vi "Read menu reference.vi"(8 "error in (no error)":errorcluster, 11 "Waveform_Task in":refnum<class "Waveform_Task.lvclass">) -> (0 "error out":errorcluster, 2 "menu reference":refnum<k9>, 3 "Waveform_Task out":refnum<class "Waveform_Task.lvclass">)   [LabVIEW 2025, in "Waveform_Task.lvlib" / "Waveform_Task.lvclass"]
uses:
  Waveform_Task.lvclass
  Waveform_Task.lvclass/Waveform_Task.ctl
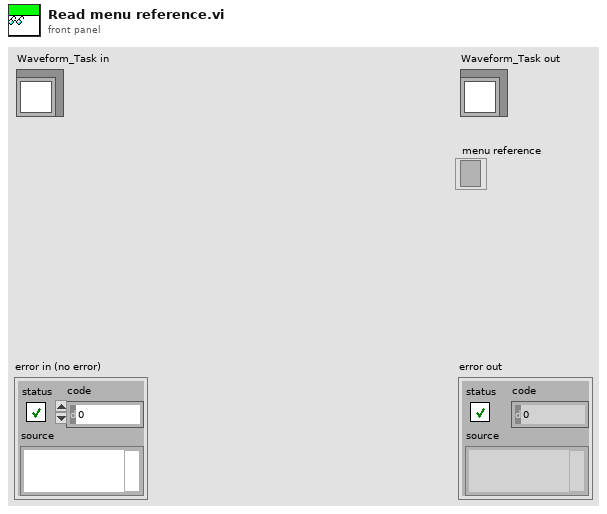
[diagram p1: front panel]
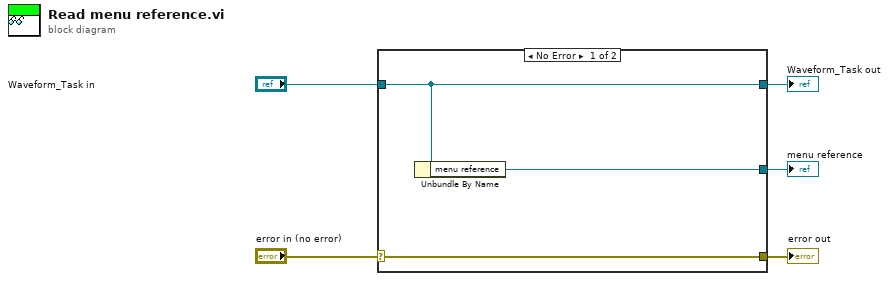
[diagram p0: block diagram]
diagram:
  n1 = case shown="No Error" "error in (no error)" {
    selector: "error in (no error)" -> [w8 w9]
    tunnel: [w8 w9] -> w4
    tunnel: [w7 w10] -> w2
    tunnel: "Waveform_Task in" -> [w7 w10]
    tunnel: [w6 _] -> w1
    frame No Error {
      n2 = Unbundle By Name(w7) -> ("menu reference"=w6:refnum<k9>)
    }
    frame Error {
    }
  }
  "error out" <- w4
  "Waveform_Task out" <- w2
  "menu reference" <- w1
